vi "HS_StopScript.vi"(8 "error in":errorcluster, 9 "Console In":string, 11 "VISA Refnum in":refnum<visa-resource-name>) -> (0 "error out":errorcluster, 1 "Console Out":string, 2 "Tx for stopping code":string, 3 "VISA Refnum out":refnum<visa-resource-name>)   [LabVIEW 2019]
panel:
  out "Reply":string
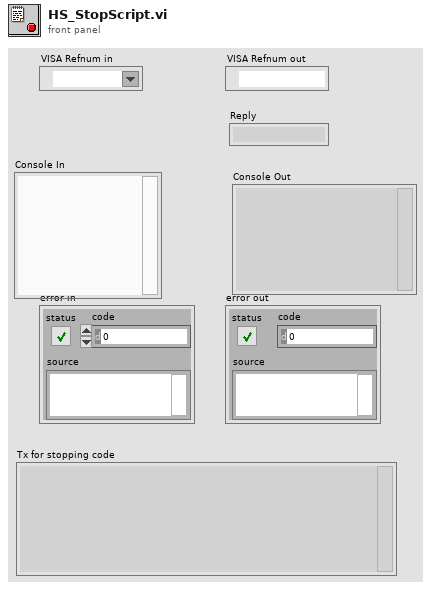
[diagram p1: front panel]
types:
  T1 = cluster{"Before":u8, "After":u8, "Send as 1 block?":bool}
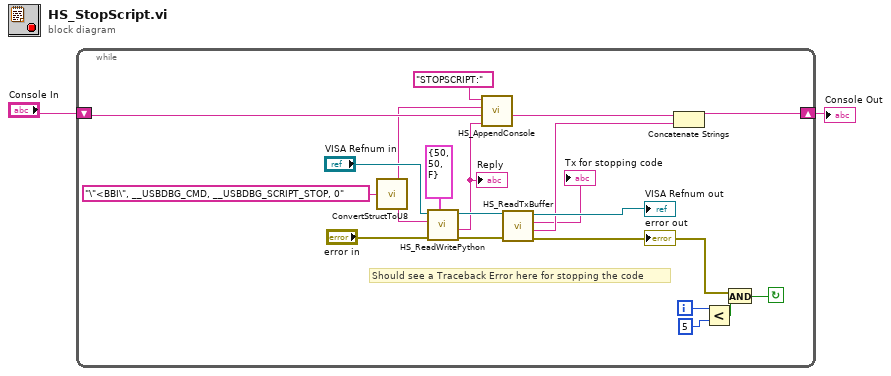
[diagram p0: block diagram]
diagram:
  n1 = while {
    shift-right: [w14] -> w1
    shift-left: "Console In" -> [w7]
    i -> [w20]
    stop <- w16 continue-if-true
    # "Should see a Traceback Error here for stopping the code"
    n2 = call <userlib>:"ConvertStructToU8.vi"("struct"="\"<BBI\", __USBDBG_CMD, __USBDBG_SCRIPT_STOP, 0" ("write buffer")) -> ("Binary"=w4:string)
    n3 = call <userlib>:"HS_ReadWritePython.vi"("Timeouts (ms)"=T1 {"Before"=50, "After"=50, "Send as 1 block?"=FALSE}, "error in"="error in", "Write"=w4, "VISA in"="VISA Refnum in") -> ("error out"=w10:errorcluster, "Console Out"=w8:string, "VISA out"=w11:refnum<visa-resource-name>)  [unwired: 2 in, 3 out]
    "Reply" <- w8
    n4 = call <userlib>:"HS_AppendConsole.vi"("Reply"=w8, "Console in"=w7, "Send"=w4, "Command"="STOPSCRIPT:") -> ()  [unwired: 7 in, 1 out]
    n5 = call <userlib>:"HS_ReadTxBuffer.vi"("error in"=w10, "VISA Refnum in"=w11) -> ("error out"=w17:errorcluster, "Console Out"=w15:string, "Tx Buffer"=→"Tx for stopping code":string, "VISA Refnum out"=→"VISA Refnum out":refnum<visa-resource-name>)  [unwired: 6 in]
    "error out" <- w17
    n6 = Concatenate Strings(w7, w15) -> (w14:string)
    n7 = Less?(x=w20, y=5) -> (x < y?=w18:bool)
    n8 = And(x=w17, y=w18) -> (x .and. y?=w16:bool)
  }
  "Console Out" <- w1
